vi "env_read_data.vi"(8 "error in":errorcluster, 9 "Input parameters":T2, 10 "State":T3, 11 "Stop signal":T5) -> (0 "error out":errorcluster, 2 "Plot data out":T4, 3 "channel":T1)   [LabVIEW 2020]
doc: "Reads out the environmental sensors."
uses:
  <extravilib>/ChannelInstances/Tag-bool/))Channel.ctl
  <extravilib>/ChannelInstances/Tag-a[.](c(a[.](stamp),a[.](dbl)))/))Channel.ctl
  <extravilib>/ChannelInstances/Tag-str/))Channel.ctl
  <extravilib>/ChannelInstances/Tag-t'input_params.ctl'/))Channel.ctl
  input_params.ctl
  <extravilib>/ChannelInstances/Tag-t'data_env.ctl'/))Channel.ctl
  data_env.ctl
  <extravilib>/ChannelInstances/Tag-t'input_params.ctl'/Read With Abort.vi
  <extravilib>/ChannelInstances/Tag-str/Read With Abort.vi
  <extravilib>/ChannelInstances/Tag-a[.](c(a[.](stamp),a[.](dbl)))/Write With Abort.vi
  <extravilib>/ChannelInstances/Tag-t'data_env.ctl'/Write With Abort.vi
  <extravilib>/ChannelInstances/Tag-bool/Read With Abort.vi
  <extravilib>/ChannelInstances/Tag-t'input_params.ctl'/EndpointRead.vi
  <extravilib>/ChannelInstances/Tag-str/EndpointRead.vi
  <extravilib>/ChannelInstances/Tag-a[.](c(a[.](stamp),a[.](dbl)))/Endpoint.vi
  <extravilib>/ChannelInstances/Tag-t'data_env.ctl'/Endpoint.vi
  <extravilib>/ChannelInstances/Tag-bool/EndpointRead.vi
  <extravilib>/ChannelInstances/Tag-bool.lvlib
  <extravilib>/ChannelInstances/Tag-a[.](c(a[.](stamp),a[.](dbl))).lvlib
  <extravilib>/ChannelInstances/Tag-str.lvlib
  <extravilib>/ChannelInstances/Tag-t'input_params.ctl'.lvlib
  <extravilib>/ChannelInstances/Tag-t'data_env.ctl'.lvlib
panel:
  out "Probecard temperature":dbl
  out "Probecard humidity":dbl
  out "Switchboard Handle":u32
  out "Ask switchboard?":bool
  out "Matrix temperature":dbl
  out "Matrix humidity":dbl
  in  "Sample period (s)":sgl=2.0
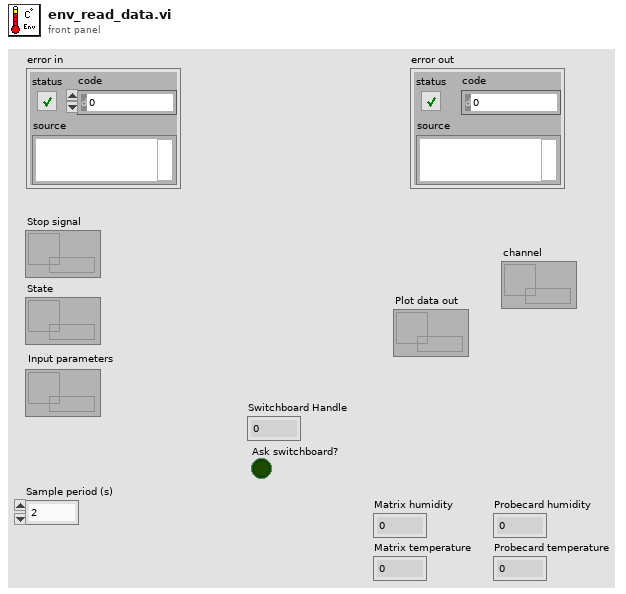
[diagram p1: front panel]
types:
  T1 = typedef "Tag-t'data_env.ctl'.lvlib/))Channel.ctl" = refnum<queue>
  T2 = typedef "Tag-t'input_params.ctl'.lvlib/))Channel.ctl" = refnum<queue>
  T3 = typedef "Tag-str.lvlib/))Channel.ctl" = refnum<queue>
  T4 = typedef "Tag-a[.](c(a[.](stamp),a[.](dbl))).lvlib/))Channel.ctl" = refnum<queue>
  T5 = typedef "Tag-bool.lvlib/))Channel.ctl" = refnum<queue>
  T6 = typedef "data_env.ctl" = cluster{"Temp. Sensirion":dbl, "Hum. Sensirion":dbl, "Temp. Switch Matrix":dbl, "Hum. Switch Matrix":dbl, "Temp. Probecard":dbl, "Hum. Probecard":dbl}
  T7 = typedef "input_params.ctl" = cluster{"Measurement type":enum16{"IV", "CV", "Debug", "Test_contact"}, "Sensor type":enum16{"HPK_6in_135ch", "HPK_8in_271ch", "IFX_8in_256ch", "Diode", "HPK_6in_239ch", "Full_Matrix", "HPK_8in_271ch_full", "LumiCal", "HPK_8in_444ch", "HPK_8in_198ch_2019", "HPK_8in_MGW_LD_full", "HPK_8in_MGW_LD_a_type_top", "HPK_8in_MGW_LD_a_type_bottom", "HPK_8in_MGW_LD_b_type_left", "HPK_8in_MGW_LD_b_type_right", "HPK_8in_MGW_LD_c_type_left", "HPK_8in_MGW_LD_c_type_right", "HPK_8in_MGW_HD_full", "HPK_8in_MGW_HD_a_type_top", "HPK_8in_MGW_HD_a_type_bottom", "HPK_8in_MGW_HD_b_type_left", "HPK_8in_MGW_HD_b_type_right", "HPK_8in_MGW_HD_c_type_left", "HPK_8in_MGW_HD_c_type_right", "CALICE_6in_256ch"}, "Identifier":string, "Open after execution?":bool, "Plot after execution?":bool, "Display channel":i32, "Voltage Delay (s)":dbl, "Switch Delay (s)":dbl, "VISA resource name source":refnum<visa-resource-name>, "VISA resource name DMM":refnum<visa-resource-name>, "VISA resource name LCR":refnum<visa-resource-name>, "Compliance  Level (A)":dbl, "Voltage Limit (V)":dbl, "Data storage location":string, "Scan voltages":string, "Use source as DMM?":bool, "LCR signal frequenzy (Hz)":dbl, "DMM device":enum16{"Keithley2001", "Keithley2450", "Keithley2410", "Keithley6485", "Keithley6487", "Keithley6517"}, "Sampling number":i32, "Use env. sensors on":enum16{"Sensirion sht1x/7x", "Switch Matrix", "Probecard"}, "Switchboard Handle":u32, "Use Switchboard":bool, "LCR signal voltage (V)":dbl, "Repeat":i32, "Scan voltages IV":string, "Scan voltages CV":string, "Hex pad numbers?":bool, "Set measurement type":enum16{"IV", "CV", "Debug", "Test_contact", "IV+CV"}, "Custom pad scan":string, "IV voltage Delay (s)":dbl, "CV voltage Delay (s)":dbl, "Needle measurement?":bool, "Comments":string, "LCR signal frequenzy (kHz)":dbl, "Compliance  Level (uA)":dbl, "Open Correction Array":dbl[][], "Current set voltage":dbl, "Last set voltage":dbl, "Current channel":i32, "Last OpenCorrection index":i32, "Total curr/vltg every x steps":i32, "Current channel iteration":i32, "No CV corrections":bool, "Mapfile":string, "Corrfile":string, "IV voltage file":path, "CV voltage file":path, "IV Switch Delay (s)":dbl, "CV Switch Delay (s)":dbl, "Invert polarity":bool, "Set debug dirs":bool, "Is n on p":bool, "Source interlock?":bool, "Voltage file used?":bool, "Pad mask":string, "Mask pad above (uA)":dbl, "LCR device":enum16{"LCR_E4980", "AGILENT_4263X"}, "Source device":enum16{"Source_2410", "Source_6487"}, "HexPlot binary path":string, "PadReductionFactor":dbl, "Temperature degC":string, "Fluence [neq]":string, "Annealing [min]":string}
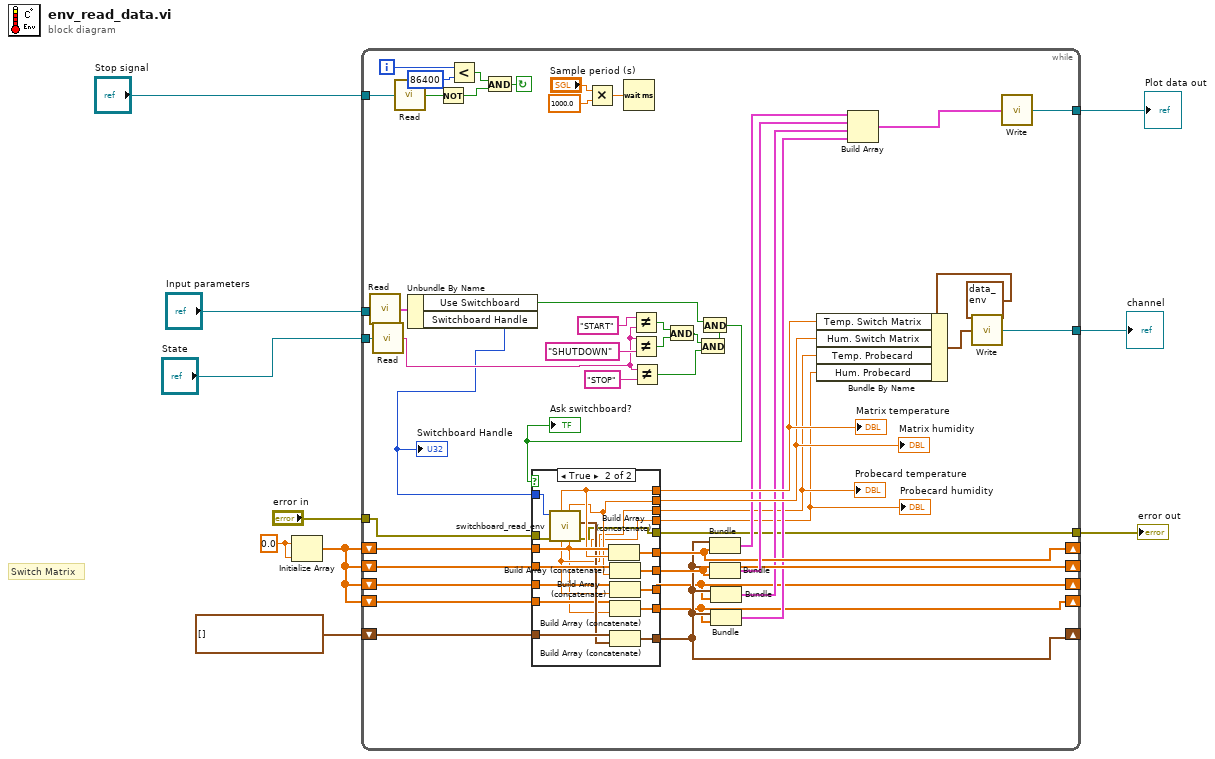
[diagram p0: block diagram]
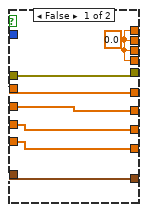
[diagram p2: hidden frame]
diagram:
  w7 = 0.0
  # "Switch Matrix"
  n1 = Initialize Array(w7, w7) -> (w5:dbl[])
  n2 = while {
    tunnel: "Stop signal" -> [w56]
    tunnel: [w11] -> w1
    tunnel: [w51] -> w9
    tunnel: "State" -> [w45]
    shift-right: [w30] -> _
    shift-left: w5 -> [w42]
    shift-right: [w32] -> _
    shift-left: w5 -> [w33]
    shift-right: [w22] -> _
    shift-left: timestamp[] [] -> [w31]
    shift-right: [w19] -> _
    shift-left: w5 -> [w24]
    shift-right: [w18] -> _
    shift-left: w5 -> [w23]
    tunnel: "error in" -> [w15]
    tunnel: [w14] -> w3
    tunnel: "Input parameters" -> [w13]
    i -> [w52]
    stop <- w57 continue-if-true
    n3 = call <extravilib>:"Read.vi"("channel"=w13) -> ("element"=w12:T7)  [unwired: 1 in, 1 out]
    n4 = call <extravilib>:"Read.vi"("channel"=w45) -> ("element"=w27:string)  [unwired: 1 in, 1 out]
    n5 = call <extravilib>:"Read.vi"("channel"=w56) -> ("element"=w55:bool)  [unwired: 1 in, 1 out]
    n6 = Unbundle By Name(w12) -> ("Use Switchboard"=w26:bool, "Switchboard Handle"=w25:u32)
    "Switchboard Handle" <- w25
    n7 = Not(x=w55) -> (.not. x?=w60:bool)
    n8 = Less?(x=w52, y=86400) -> (x < y?=w59:bool)
    n9 = And(x=w59, y=w60) -> (x .and. y?=w57:bool)
    n10 = Multiply(x="Sample period (s)", y=sgl 1000.0) -> (x*y=w50:sgl)
    n11 = Wait (ms)(milliseconds to wait=w50) -> ()  [unwired: 1 out]
    n12 = Not Equal?(x="START", y=w27) -> (x != y?=w46:bool)
    n13 = Not Equal?(x=w27, y="SHUTDOWN") -> (x != y?=w47:bool)
    n14 = Not Equal?(x=w27, y="STOP") -> (x != y?=w28:bool)
    n15 = And(x=w46, y=w47) -> (x .and. y?=w37:bool)
    n16 = And(x=w37, y=w28) -> (x .and. y?=w36:bool)
    n17 = And(x=w26, y=w36) -> (x .and. y?=w29:bool)
    "Ask switchboard?" <- w29
    n18 = case shown="True" w29 {
      tunnel: w25 -> [_ w85]
      tunnel: w42 -> [w65 w84]
      tunnel: [w62 w80] -> w41
      tunnel: [w62 w79] -> w40
      tunnel: w33 -> [w66 w83]
      tunnel: [w66 w77] -> w32
      tunnel: w31 -> [w67 w82]
      tunnel: [w67 w81] -> w22
      tunnel: [w65 w76] -> w30
      tunnel: w24 -> [w64 w72]
      tunnel: w23 -> [w63 w73]
      tunnel: [w64 w75] -> w19
      tunnel: [w63 w74] -> w18
      tunnel: [w62 w71] -> w17
      tunnel: [w62 w70] -> w16
      tunnel: w15 -> [w61 w69]
      tunnel: [w61 w68] -> w14
      frame False {
        w62 = 0.0 ("Matrix temperature")
      }
      frame True {
        n19 = call "switchboard_read_env.vi"("error in"=w69, "Handle"=w85) -> ("error out"=w68:errorcluster, "current time"=w78:timestamp, "Probecard humidity"=w70:dbl, "Matrix humidity"=w79:dbl, "Probecard temperature"=w71:dbl, "Matrix temperature"=w80:dbl)  [unwired: 3 in, 1 out]
        n20 = Build Array (concatenate)(w84, w80) -> (w76:dbl[])
        n21 = Build Array (concatenate)(w83, w79) -> (w77:dbl[])
        n22 = Build Array (concatenate)(w72, w71) -> (w75:dbl[])
        n23 = Build Array (concatenate)(w73, w70) -> (w74:dbl[])
        n24 = Build Array (concatenate)(w82, w78) -> (w81:timestamp[])
      }
    }
    "Matrix humidity" <- w40
    "Matrix temperature" <- w41
    "Probecard humidity" <- w16
    "Probecard temperature" <- w17
    n25 = Bundle(w22, w30) -> (w39:cluster{timestamp[], dbl[]})  [unwired: 1 out]
    n26 = Bundle(w22, w32) -> (w34:cluster{timestamp[], dbl[]})  [unwired: 1 out]
    n27 = Bundle(w22, w19) -> (w21:cluster{timestamp[], dbl[]})  [unwired: 1 out]
    n28 = Bundle(w22, w18) -> (w20:cluster{timestamp[], dbl[]})  [unwired: 1 out]
    n29 = Bundle By Name(cluster=T6 {"Temp. Sensirion"=0.01, "Hum. Sensirion"=0.01, "Temp. Switch Matrix"=0.01, "Hum. Switch Matrix"=0.01, "Temp. Probecard"=0.01, "Hum. Probecard"=0.01} ("Cluster"), "Temp. Switch Matrix"=w41, "Hum. Switch Matrix"=w40, "Temp. Probecard"=w17, "Hum. Probecard"=w16) -> (w54:T6)
    n30 = Build Array(w39, w34, w21, w20) -> (w35:cluster{timestamp[], dbl[]}[])
    n31 = call <extravilib>:"Write.vi"("element"=w54) -> ("channel"=w11:T1)  [unwired: 1 out]
    n32 = call <extravilib>:"Write.vi"("element"=w35) -> ("channel"=w51:T4)  [unwired: 1 out]
  }
  "Plot data out" <- w9
  "error out" <- w3
  "channel" <- w1
